vi "uStringManipulation_1-to-1_Map_Set.vi"(8 "error in (no error)":errorcluster, 10 "Mapping":string[][](array[string]), 11 "1-to-1_map in":refnum<class "1-to-1_map.lvclass">) -> (0 "error out":errorcluster, 3 "1-to-1_map out":refnum<class "1-to-1_map.lvclass">)   [LabVIEW 2023, in "uLib.lvlib" / "1-to-1_map.lvclass"]
doc: "Use to enter the map as a 2D array. The first column is the key and the second column is the destination translation."
uses:
  1-to-1_map.lvclass
  1-to-1_map.lvclass/1-to-1_map.ctl
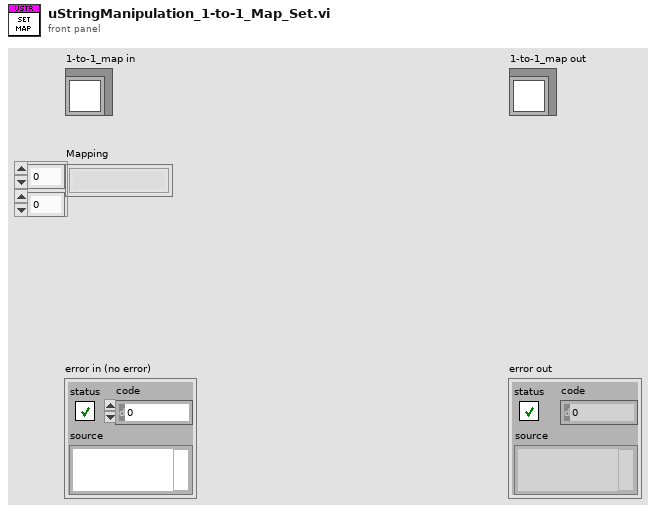
[diagram p1: front panel]
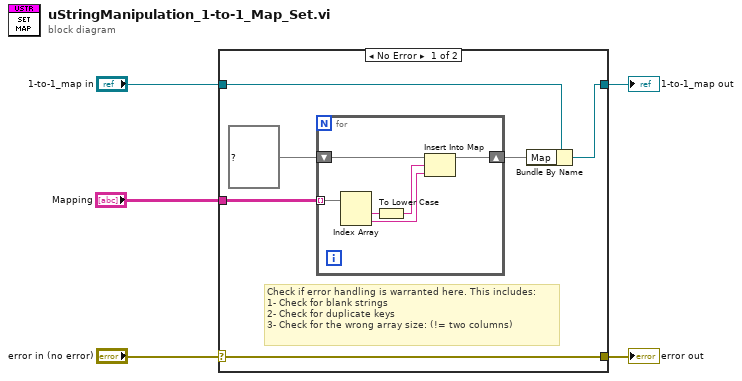
[diagram p0: block diagram]
diagram:
  n1 = case shown="No Error" "error in (no error)" {
    selector: "error in (no error)" -> [w11 w18]
    tunnel: [w11 w18] -> w4
    tunnel: [w9 w19] -> w2
    tunnel: "1-to-1_map in" -> [w10 w19]
    tunnel: "Mapping" -> [w8 _]
    frame No Error {
      # "Check if error handling is warranted here. This includes:\n1- Check for blank strings\n2- Check for duplicate keys\n3- Check for the wrong array size: (!= two columns)"
      n2 = for {
        tunnel: w8 -> [w17] mode=indexing
        shift-right: [w13] -> w6
        shift-left: map{string, string} {} ("Map") -> [w12]
        n3 = Index Array(array=w17) -> (element #1=w15:string, element #2=w16:string)  [unwired: 2 in]
        n4 = To Lower Case(string=w15) -> (all lower case string=w14:string)
        n5 = Insert Into Map(map in=w12, key=w14, value=w16) -> (map out=w13:map{string, string})  [unwired: 2 out]
      }
      n6 = Bundle By Name(cluster=w10, "Map"=w6) -> (w9:refnum<class "1-to-1_map.lvclass">)
    }
    frame Error {
    }
  }
  "error out" <- w4
  "1-to-1_map out" <- w2
